vi "题目2.vi"() -> ()   [LabVIEW 2017]
panel:
  out "数值 2":dbl
  out "数值":dbl
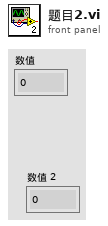
[diagram p1: front panel]
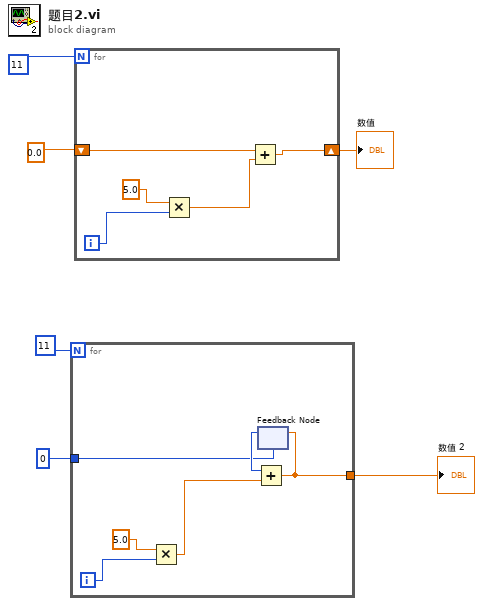
[diagram p0: block diagram]
diagram:
  n1 = for {
    N: 11 -> [_]
    tunnel: [w9] -> w5
    tunnel: 0 -> [w7]
    i -> [w12]
    n2 = Multiply(x=5.0, y=w12) -> (x*y=w10:dbl)
    n3 = feedback #1(w7) -> (w8:i32)
    n4 = Add(x=w8, y=w10) -> (x+y=w9:dbl)
    n5 = feedback-in #1(w9) -> ()
  }
  "数值 2" <- w5
  n6 = for {
    N: 11 -> [_]
    shift-right: [w16] -> w6
    shift-left: 0.0 -> [w13]
    i -> [w17]
    n7 = Multiply(x=5.0, y=w17) -> (x*y=w15:dbl)
    n8 = Add(x=w13, y=w15) -> (x+y=w16:dbl)
  }
  "数值" <- w6
